vi "getCalibratedPhase.vi"(8 "error in (no error)":errorcluster, 11 "rf in":refnum<class "rf.lvclass">) -> (0 "error out":errorcluster, 2 "calibratedPhase":dbl, 3 "rf out":refnum<class "rf.lvclass">)   [LabVIEW 2009, in "Tools.lvlib" / "Scripting.lvlib" / "rf.lvclass"]
uses:
  rf.lvclass
  rf.lvclass/rf.ctl
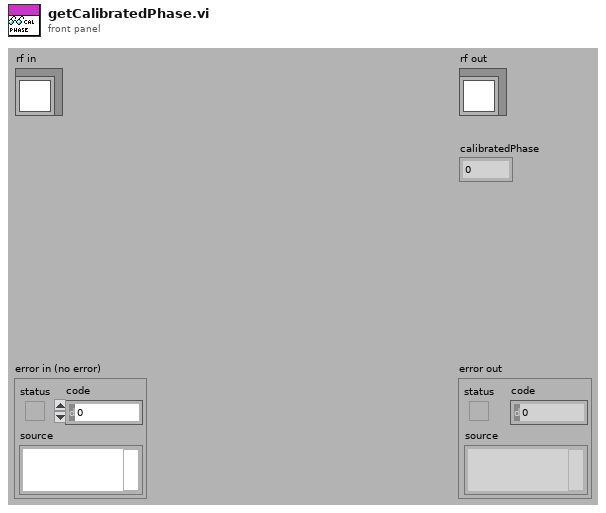
[diagram p1: front panel]
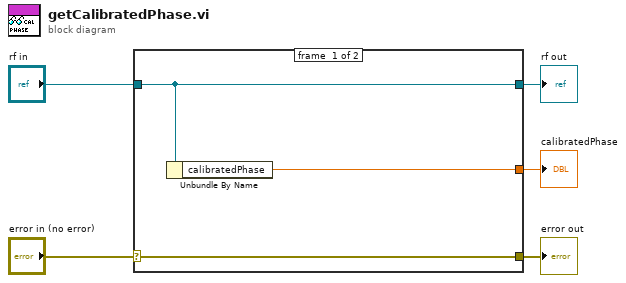
[diagram p0: block diagram]
diagram:
  n1 = case shown="No Error" "error in (no error)" {
    selector: "error in (no error)" -> [w8 w9]
    tunnel: [w8 w9] -> w4
    tunnel: [w7 w10] -> w2
    tunnel: "rf in" -> [w7 w10]
    tunnel: [w6 _] -> w1
    frame #0 {
      n2 = Unbundle By Name(w7) -> ("calibratedPhase"=w6:dbl)
    }
    frame #1 {
    }
  }
  "error out" <- w4
  "rf out" <- w2
  "calibratedPhase" <- w1
